vi "Find Item Locations by Path.vi"(5 "Insertion point if not found":bool, 6 "Only return first found":bool, 7 "Path":string, 8 "error in (no error)":errorcluster, 10 "Offset":i32, 11 "JSON":string) -> (0 "error out":errorcluster, 1 "Items":T1[](array[typedef]))   [LabVIEW 2017, in "JSONtext.lvlib"]
uses:
  JSONtext.lvlib
  Parsing/Found Items.ctl
  Parsing/Parsing State.ctl
  <vilib>/JDP Science/JDP Science Common Utilities/Trim Whitespace__JDP.vi
  Parsing/Advance past whitespace and comma.vi
  Parsing/Advance past next JSON Value (inlined COPY).vi
  Parsing/Advance past Item Name.vi
  Parsing/Advance past next JSON Scaler.vi
  Parsing/Match Pattern.vi
  support/Quote and Escape JSON string.vi
  Parsing/Advance past String.vi
  String Subset.vi
  Parsing/Advance past Number.vi
  support/quote and escape json string 2.vi
  Parsing/Advance past Array.vi
  Parsing/Advance past Object.vi
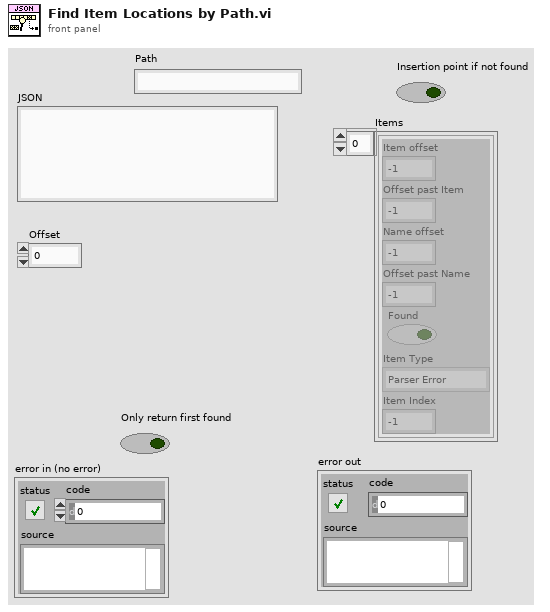
[diagram p1: front panel]
types:
  T1 = typedef "JSONtext.lvlib/Found Items.ctl" = cluster{"Item offset":i32, "Offset past Item":i32, "Name offset":i32, "Offset past Name":i32, "Found":bool, "Item Type":T2, "Item Index":i32}
  T2 = typedef "JSONtext.lvlib/Parsing State.ctl" = enum16{"Parser Error", "Object", "Array", "String", "Number/Other", "Leading Whitespace", "Object end", "Array end", "Value end"}
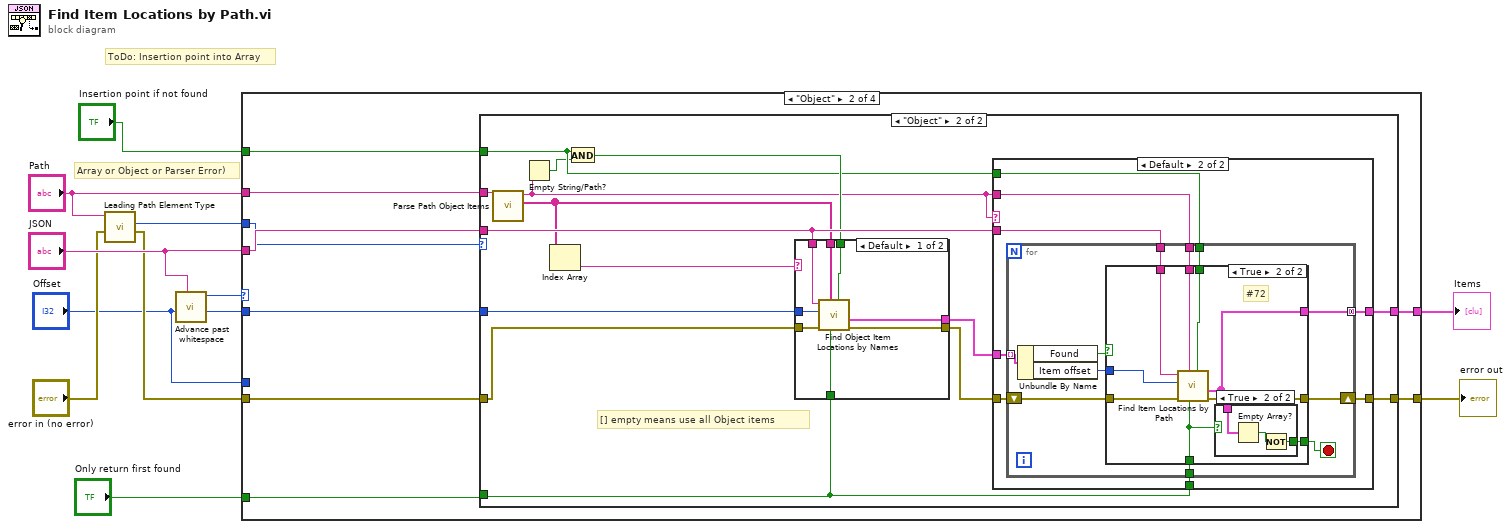
[diagram p0: block diagram]
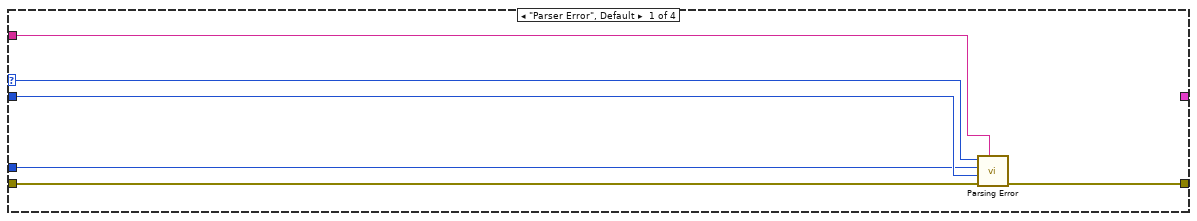
[diagram p2: hidden frame]
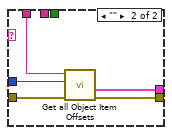
[diagram p4: hidden frame]
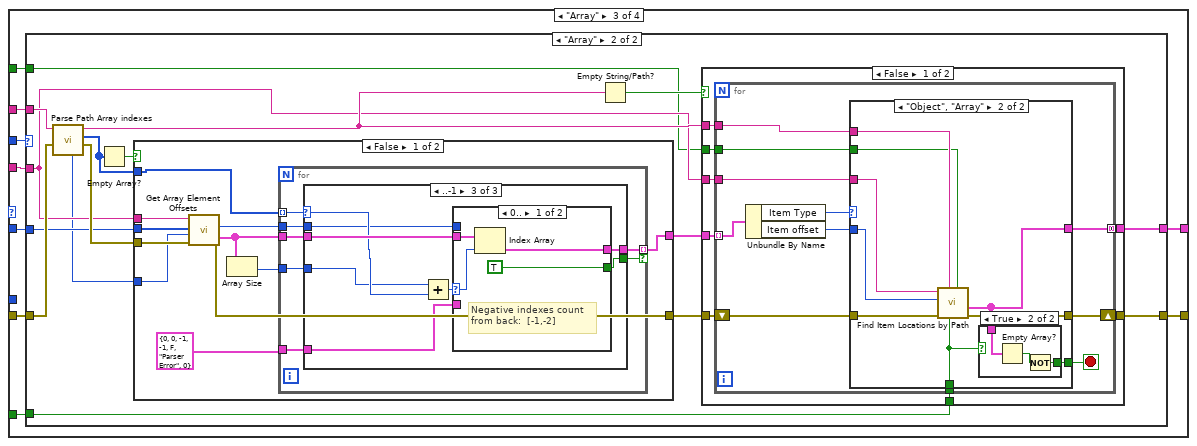
[diagram p8: hidden frame]
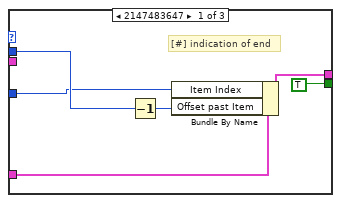
[diagram p10: hidden frame]
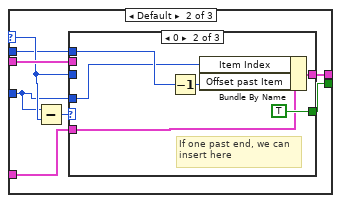
[diagram p11: hidden frame]
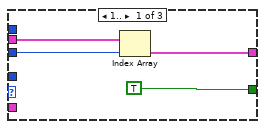
[diagram p12: hidden frame]
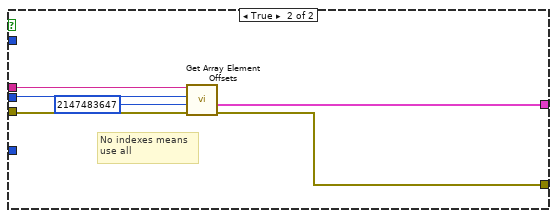
[diagram p15: hidden frame]
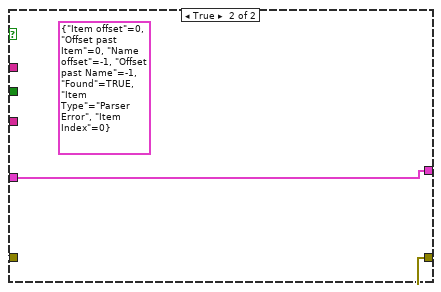
[diagram p18: hidden frame]
diagram:
  # "Array or Object or Parser Error)"
  # "ToDo: Insertion point into Array"
  n1 = call "Leading Path Element Type.vi"("error in (no error)"="error in (no error)", "Path"="Path") -> ("error out"=w4:errorcluster, "Path Element Type (Array or Object or Parser Error)"=w1:T2)  [unwired: 8 in]
  n2 = call "Advance past whitespace.vi"("JSON"="JSON", "Offset"="Offset") -> ("Offset of first non-whitespace"=w10:i32, "Parser State"=w3:T2)  [unwired: 8 in]
  n3 = case shown="\"Object\"" w3 {
    selector: w3 -> [w16 _ _ _]
    tunnel: [_ w26 w98 _] -> w12
    tunnel: w4 -> [w18 w24 w95 w211]
    tunnel: [w17 w27 w99 w211] -> w9
    tunnel: "Path" -> [_ w23 w96 _]
    tunnel: "Only return first found" -> [_ w21 w97 _]
    tunnel: "Insertion point if not found" -> [_ w20 w91 _]
    tunnel: w10 -> [w15 w22 w94 _]
    tunnel: "JSON" -> [w14 w25 w93 _]
    tunnel: "Offset" -> [w13 _ _ _]
    tunnel: w1 -> [_ w19 w92 _]
    frame "Parser Error", Default {
      n4 = call "Parsing Error.vi"("JSON"=w14, "error in (no error)"=w18, "Offset past match"=w15, "Value start"=w13, "State"=w16) -> ("error out"=w17:errorcluster)  [unwired: 6 in]
    }
    frame "Object" {
      n5 = case shown="\"Object\"" w19 {
        tunnel: [w28 w43] -> w27
        tunnel: [_ w42] -> w26
        tunnel: w25 -> [_ w41]
        tunnel: w24 -> [w28 w40]
        tunnel: w23 -> [_ w39]
        tunnel: w22 -> [_ w38]
        tunnel: w21 -> [_ w33]
        tunnel: w20 -> [_ w31]
        frame Default {
        }
        frame "Object" {
          # "[] empty means use all Object items"
          n6 = call "Parse Path Object Items.vi"("Path with leading Object element"=w39) -> ("<JSON>items names"=w35:string[], "Rest or Path"=w29:string)  [unwired: 7 in, 2 out]
          n7 = Empty String/Path?(string/path=w29) -> (empty?=w30:bool)
          n8 = Index Array(array=w35) -> (element=w34:string)  [unwired: 1 in]
          n9 = And(x=w31, y=w30) -> (x .and. y?=w32:bool)
          n10 = case shown="Default" w34 {
            tunnel: w41 -> [w51 w56]
            tunnel: w40 -> [w50 w54]
            tunnel: w38 -> [w49 w55]
            tunnel: w35 -> [w48 _]
            tunnel: [w47 w53] -> w37
            tunnel: [w46 w52] -> w36
            tunnel: w33 -> [w45 _]
            tunnel: w32 -> [w44 _]
            frame Default {
              n11 = call "Find Object Item Locations by Names.vi"("Insertion point if not found"=w44, "Only return first found"=w45, "Item Names <JSON>"=w48, "error in (no error)"=w50, "Object Offset"=w49, "JSON"=w51) -> ("error out"=w47:errorcluster, "Items"=w46:T1[])  [unwired: 4 in]
            }
            frame "" {
              n12 = call "Get all Object Item Offsets.vi"("error in (no error)"=w54, "Offset"=w55, "JSON"=w56) -> ("error out"=w53:errorcluster, "Items"=w52:T1[])  [unwired: 6 in, 1 out]
            }
          }
          n13 = case shown="Default" w29 {
            tunnel: [w57 w66] -> w43
            tunnel: [w58 w65] -> w42
            tunnel: w41 -> [_ w64]
            tunnel: w29 -> [_ w63]
            tunnel: w37 -> [w57 w62]
            tunnel: w36 -> [w58 w61]
            tunnel: w33 -> [_ w60]
            tunnel: w31 -> [_ w59]
            frame "" {
            }
            frame Default {
              n14 = for {
                tunnel: [w76] -> w65 mode=concatenating
                tunnel: w64 -> [w75]
                tunnel: w63 -> [w74]
                tunnel: w61 -> [w72] mode=indexing
                shift-right: [w77] -> w66
                shift-left: w62 -> [w73]
                tunnel: w60 -> [w69]
                tunnel: w59 -> [w67]
                stop <- w68 stop-if-true
                n15 = Unbundle By Name(w72) -> ("Found"=w71:bool, "Item offset"=w70:i32)
                n16 = case shown="True" w71 {
                  tunnel: [w78 w87] -> w77
                  tunnel: [_ w81] -> w76
                  tunnel: w75 -> [_ w86]
                  tunnel: w74 -> [_ w85]
                  tunnel: w73 -> [w78 w84]
                  tunnel: w70 -> [_ w83]
                  tunnel: w69 -> [_ w82]
                  tunnel: [_ w80] -> w68
                  tunnel: w67 -> [_ w79]
                  frame False {
                  }
                  frame True {
                    # "#72"
                    n17 = call "Find Item Locations by Path.vi"("Insertion point if not found"=w79, "Only return first found"=w82, "Path"=w85, "error in (no error)"=w84, "Offset"=w83, "JSON"=w86) -> ("error out"=w87:errorcluster, "Items"=w81:T1[])  [unwired: 4 in]
                    n18 = case shown="True" w82 {
                      tunnel: w81 -> [_ w90]
                      tunnel: [_ w88] -> w80
                      frame False {
                      }
                      frame True {
                        n19 = Empty Array?(array=w90) -> (empty?=w89:bool)
                        n20 = Not(x=w89) -> (.not. x?=w88:bool)
                      }
                    }
                  }
                }
              }
            }
          }
        }
      }
    }
    frame "Array" {
      n21 = case shown="\"Array\"" w92 {
        tunnel: [w100 w116] -> w99
        tunnel: [_ w115] -> w98
        tunnel: w97 -> [_ w114]
        tunnel: w96 -> [_ w113]
        tunnel: w95 -> [w100 w112]
        tunnel: w94 -> [_ w105]
        tunnel: w93 -> [_ w104]
        tunnel: w91 -> [_ w101]
        frame "Parser Error", Default {
        }
        frame "Array" {
          n22 = call "Parse Path Array indexes.vi"("error in (no error)"=w112, "Path with leading Array element"=w113) -> ("error out"=w106:errorcluster, "Indexes (empty means use all)"=w107:i32[], "Rest or Path"=w111:string, "Max Index to parse"=w102:i32)  [unwired: 6 in]
          n23 = Empty Array?(array=w107) -> (empty?=w109:bool)
          n24 = case shown="False" w109 {
            tunnel: [w127 w172] -> w108
            tunnel: w107 -> [w119 _]
            tunnel: w106 -> [w125 w174]
            tunnel: w105 -> [w124 w175]
            tunnel: w104 -> [w123 w176]
            tunnel: [w122 w173] -> w103
            tunnel: w102 -> [w118 _]
            frame False {
              n25 = call "Get Array Element Offsets.vi"("error in (no error)"=w125, "Max Index"=w118, "Offset"=w124, "JSON"=w123) -> ("error out"=w122:errorcluster, "Elements"=w121:T1[], "Offset past Array"=w120:i32)  [unwired: 5 in]
              n26 = Array Size(array=w121) -> (size(s)=w126:i32)
              n27 = for {
                tunnel: w119 -> [w132] mode=indexing
                tunnel: w121 -> [w134]
                tunnel: [w133] -> w127 mode=indexing if=w129
                tunnel: w126 -> [w131]
                tunnel: w120 -> [w130]
                tunnel: T1 {"Item offset"=0, "Offset past Item"=0, "Name offset"=-1, "Offset past Name"=-1, "Found"=FALSE, "Item Type"=enum."Parser Error", "Item Index"=0} -> [w128]
                n28 = case shown="..-1" w132 {
                  selector: w132 -> [_ w146 w164]
                  tunnel: w134 -> [_ w148 w166]
                  tunnel: [w140 w147 w165] -> w133
                  tunnel: w131 -> [w136 w142 w160]
                  tunnel: [TRUE w145 w163] -> w129
                  tunnel: w130 -> [w139 w143 w161]
                  tunnel: w128 -> [w135 w141 w159]
                  frame 2147483647 {
                    # "[#] indication of end"
                    n29 = Decrement(x=w139) -> (x-1=w138:i32)
                    n30 = Bundle By Name(cluster=w135, "Item Index"=w136, "Offset past Item"=w138) -> (w140:T1)
                  }
                  frame Default {
                    n31 = Subtract(x=w142, y=w146) -> (x-y=w144:i32)
                    n32 = case shown="0" w144 {
                      tunnel: w148 -> [w152 _ _]
                      tunnel: [w151 w156 _] -> w147
                      tunnel: w146 -> [w150 _ _]
                      tunnel: [TRUE TRUE _] -> w145
                      tunnel: w143 -> [_ w155 _]
                      tunnel: w142 -> [_ w153 _]
                      tunnel: w141 -> [_ w154 _]
                      frame 1.. {
                        n33 = Index Array(array=w152, index=w150) -> (element=w151:T1)
                      }
                      frame 0 {
                        # "If one past end, we can\ninsert here"
                        n34 = Decrement(x=w155) -> (x-1=w158:i32)
                        n35 = Bundle By Name(cluster=w154, "Item Index"=w153, "Offset past Item"=w158) -> (w156:T1)
                      }
                      frame Default {
                      }
                    }
                  }
                  frame ..-1 {
                    n36 = Add(x=w160, y=w164) -> (x+y=w162:i32)
                    n37 = case shown="0.." w162 {
                      selector: w162 -> [w167 _]
                      tunnel: w166 -> [w170 _]
                      tunnel: [w169 _] -> w165
                      tunnel: [TRUE _] -> w163
                      tunnel: w161 -> [_ _]
                      tunnel: w159 -> [_ _]
                      frame 0.. {
                        # "Negative indexes count\nfrom back:  [-1,-2]"
                        n38 = Index Array(array=w170, index=w167) -> (element=w169:T1)
                      }
                      frame Default {
                      }
                    }
                  }
                }
              }
            }
            frame True {
              # "No indexes means\nuse all"
              n39 = call "Get Array Element Offsets.vi"("error in (no error)"=w174, "Max Index"=2147483647, "Offset"=w175, "JSON"=w176) -> ("error out"=w173:errorcluster, "Elements"=w172:T1[])  [unwired: 5 in, 1 out]
            }
          }
          n40 = Empty String/Path?(string/path=w111) -> (empty?=w110:bool)
          n41 = case shown="False" w110 {
            tunnel: [w184 w210] -> w116
            tunnel: [w183 w209] -> w115
            tunnel: w108 -> [w182 w209]
            tunnel: w103 -> [w181 w210]
            tunnel: w104 -> [w180 _]
            tunnel: w114 -> [w179 _]
            tunnel: w111 -> [w178 _]
            tunnel: w101 -> [w177 _]
            frame False {
              n42 = for {
                tunnel: [w193] -> w183 mode=concatenating
                shift-right: [w194] -> w184
                shift-left: w181 -> [w195]
                tunnel: w178 -> [w192]
                tunnel: w182 -> [w191] mode=indexing
                tunnel: w180 -> [w189]
                tunnel: w179 -> [w187]
                tunnel: w177 -> [w185]
                stop <- w186 stop-if-true
                n43 = Unbundle By Name(w191) -> ("Item Type"=w190:T2, "Item offset"=w188:i32)
                n44 = case shown="\"Object\", \"Array\"" w190 {
                  tunnel: w195 -> [w196 w205]
                  tunnel: [w196 w204] -> w194
                  tunnel: [_ w200] -> w193
                  tunnel: w192 -> [_ w203]
                  tunnel: w189 -> [_ w202]
                  tunnel: w188 -> [_ w201]
                  tunnel: w187 -> [_ w198]
                  tunnel: [_ w199] -> w186
                  tunnel: w185 -> [_ w197]
                  frame "Parser Error", Default {
                  }
                  frame "Object", "Array" {
                    n45 = call "Find Item Locations by Path.vi"("Insertion point if not found"=w197, "Only return first found"=w198, "Path"=w203, "error in (no error)"=w205, "Offset"=w201, "JSON"=w202) -> ("error out"=w204:errorcluster, "Items"=w200:T1[])  [unwired: 4 in]
                    n46 = case shown="True" w198 {
                      tunnel: w200 -> [_ w208]
                      tunnel: [_ w206] -> w199
                      frame False {
                      }
                      frame True {
                        n47 = Empty Array?(array=w208) -> (empty?=w207:bool)
                        n48 = Not(x=w207) -> (.not. x?=w206:bool)
                      }
                    }
                  }
                }
              }
            }
            frame True {
              (unwired) T1 {"Item offset"=0, "Offset past Item"=0, "Name offset"=-1, "Offset past Name"=-1, "Found"=TRUE, "Item Type"=enum."Parser Error", "Item Index"=0}
            }
          }
        }
      }
    }
    frame "String", "Number/Other" {
      # "Not an object or Array so Path ends here\n\n--> throw error?"
    }
  }
  "Items" <- w12
  "error out" <- w9
